vi "Part 2.vi"(11 "Input":string) -> (3 "Output":i64)   [LabVIEW 2021]
uses:
  3dc34be2-a6d3-4b17-bbb5-65f4369eede6.vi
  <userlib>/_OpenG.lib/string/string.llb/Convert EOLs (String)__ogtk.vi
panel:
  out "Array":bool[][](array[boolean])
  out "Grid":string[][](array[string])
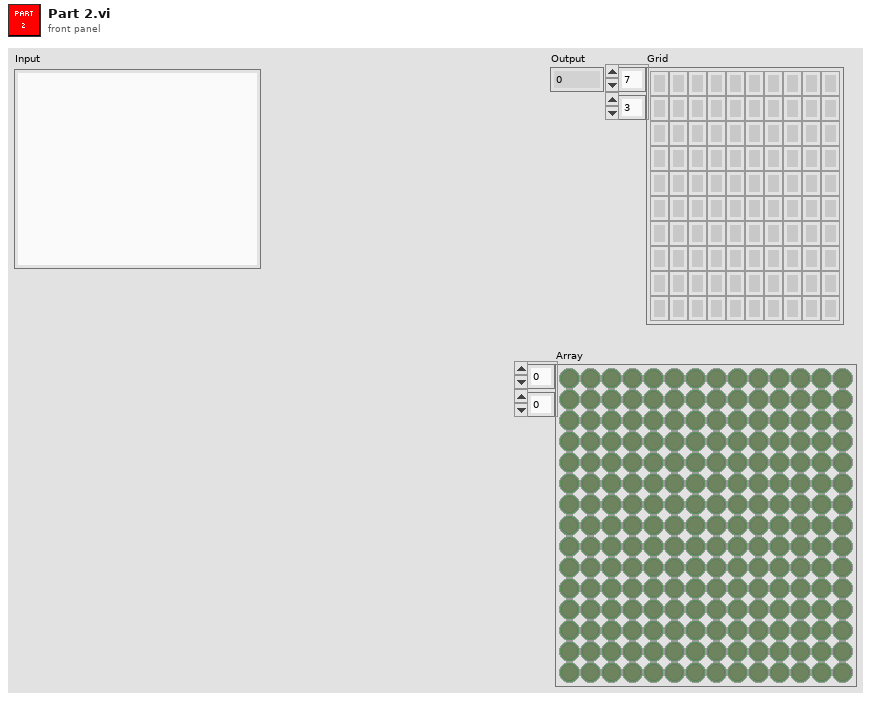
[diagram p1: front panel]
types:
  T1 = set{cluster{"row":i32, "col":i32, "dir":enum16{"right", "left", "up", "down"}}}
  T2 = cluster{"row":i32, "col":i32, "dir":enum16{"right", "left", "up", "down"}}[]
  T3 = cluster{"row":i32, "col":i32, "dir":enum16{"right", "left", "up", "down"}}
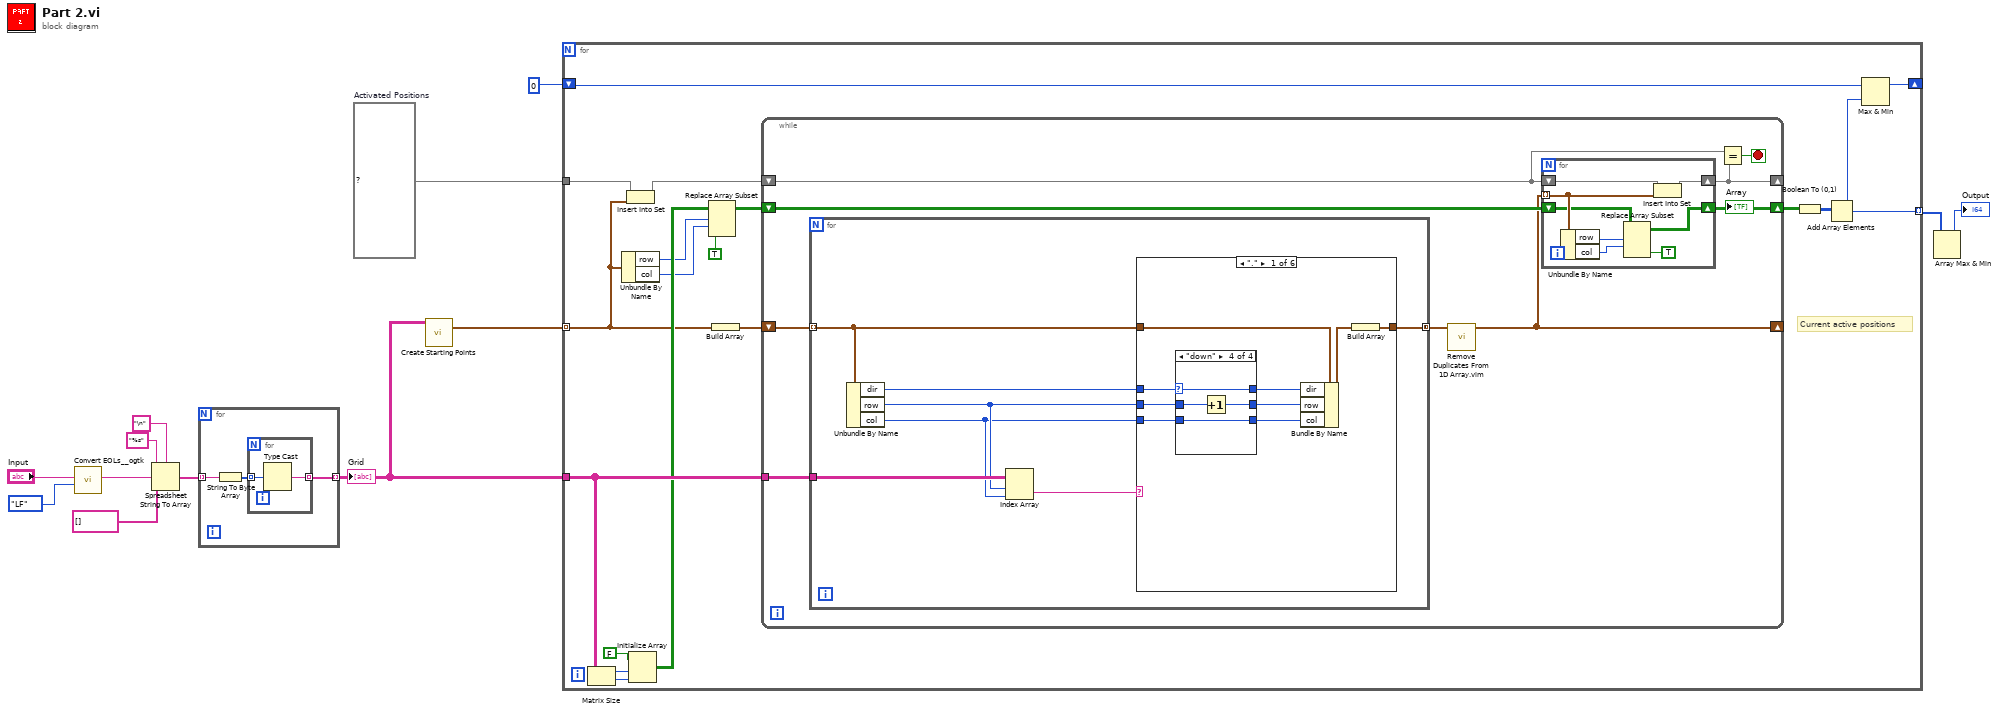
[diagram p0: block diagram]
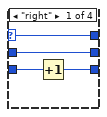
[diagram p2: hidden frame]
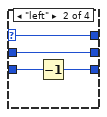
[diagram p3: hidden frame]
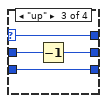
[diagram p4: hidden frame]
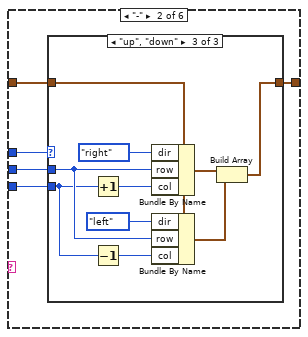
[diagram p5: hidden frame]
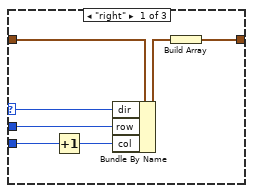
[diagram p6: hidden frame]
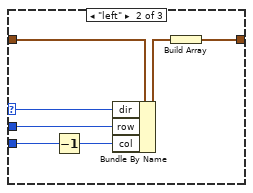
[diagram p7: hidden frame]
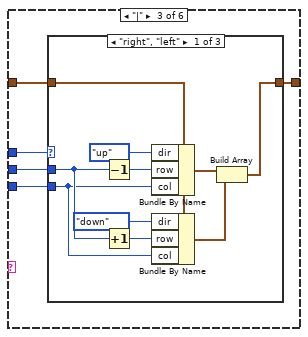
[diagram p8: hidden frame]
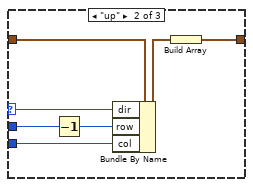
[diagram p9: hidden frame]
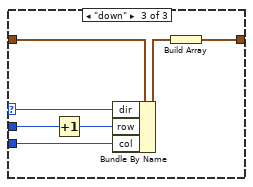
[diagram p10: hidden frame]
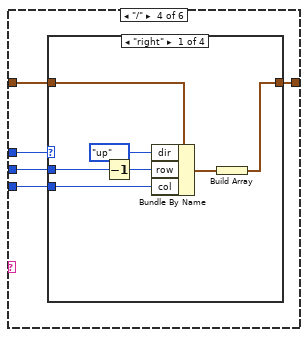
[diagram p11: hidden frame]
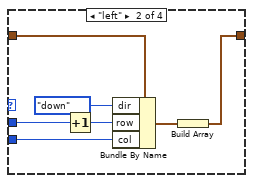
[diagram p12: hidden frame]
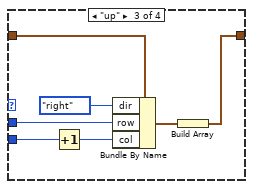
[diagram p13: hidden frame]
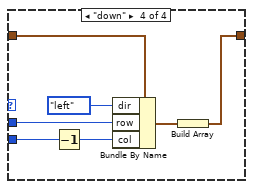
[diagram p14: hidden frame]
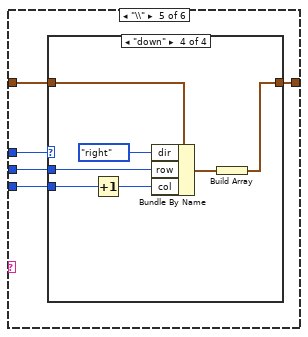
[diagram p15: hidden frame]
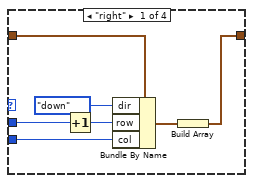
[diagram p16: hidden frame]
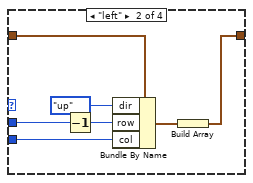
[diagram p17: hidden frame]
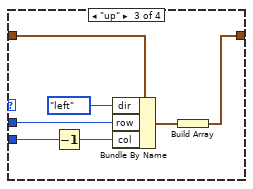
[diagram p18: hidden frame]
diagram:
  w6 = T1 {}  # Activated Positions
  n1 = call-poly <userlib>:"Convert EOLs__ogtk.vi"("Convert to:"=enum16{"CR", "LF", "CRLF"}."LF", "String in"="Input") -> ("String out"=w9:string)  [unwired: 9 in]
  n2 = Spreadsheet String To Array(delimiter (Tab)="\n", format string="%s", spreadsheet string=w9, array type (2D Dbl)=string[] []) -> (array=w7:string[])
  n3 = for {
    tunnel: w7 -> [w16] mode=indexing
    tunnel: [w14] -> w3 mode=indexing
    n4 = String To Byte Array(string=w16) -> (unsigned byte array=w15:u8[])
    n5 = for {
      tunnel: w15 -> [w18] mode=indexing
      tunnel: [w17] -> w14 mode=indexing
      n6 = Type Cast(x=w18) -> (*(type *) &x=w17:string)  [unwired: 1 in]
    }
  }
  "Grid" <- w3
  n7 = call "Create Starting Points.vi"("Grid"=w3) -> ("Starting Points"=w2:T2)  [unwired: 10 in]
  n8 = for {
    tunnel: w6 -> [w35]
    tunnel: w2 -> [w24] mode=indexing
    tunnel: w3 -> [w32]
    tunnel: [w19] -> w5 mode=indexing
    shift-right: [w21] -> _
    shift-left: 0 -> [w20]
    # "Current active positions"
    n9 = Matrix Size(0:w32) -> (1:w33:i32, 2:w31:i32)
    n10 = Unbundle By Name(w24) -> ("row"=w23:i32, "col"=w22:i32)
    n11 = Insert Into Set(10:w24, 11:w35) -> (3:w34:T1)  [unwired: 1 out]
    n12 = Initialize Array(FALSE, w33, w31) -> (w29:bool[][])
    n13 = Replace Array Subset(array=w29, new element=TRUE, index (row)=w23, index (col)=w22) -> (w28:bool[][])
    n14 = Build Array(w24) -> (w36:T2)
    n15 = while {
      shift-right: [w44] -> _
      shift-left: w34 -> [w43]
      shift-right: [w37] -> _
      shift-left: w36 -> [w42]
      tunnel: w32 -> [w40]
      shift-right: [w38] -> w26
      shift-left: w28 -> [w39]
      stop <- w45 stop-if-true
      n16 = for {
        tunnel: w42 -> [w49] mode=indexing
        tunnel: [w50] -> w41 mode=concatenating
        tunnel: w40 -> [w52]
        n17 = Unbundle By Name(w49) -> ("dir"=w48:enum16{"right", "left", "up", "down"}, "row"=w47:i32, "col"=w46:i32)
        n18 = Index Array(array=w52, index (row)=w47, index (col)=w46) -> (element=w51:string)
        n19 = case shown="\".\"" w51 {
          tunnel: w47 -> [w57 w80 w109 w138 w171 _]
          tunnel: w46 -> [w55 w79 w108 w137 w170 _]
          tunnel: w48 -> [w58 w81 w110 w139 w172 _]
          tunnel: w49 -> [w61 w82 w111 w140 w173 _]
          tunnel: [w60 w78 w107 w136 w169 _] -> w50
          frame "." {
            n20 = case shown="\"down\"" w58 {
              selector: w58 -> [w62 w66 w70 w74]
              tunnel: w57 -> [w65 w69 w72 w76]
              tunnel: w55 -> [w64 w68 w73 w77]
              tunnel: [w65 w69 w71 w75] -> w54
              tunnel: [w63 w67 w73 w77] -> w56
              tunnel: [w62 w66 w70 w74] -> w53
              frame "right" {
                n21 = Increment(x=w64) -> (x+1=w63:i32)
              }
              frame "left" {
                n22 = Decrement(x=w68) -> (x-1=w67:i32)
              }
              frame "up" {
                n23 = Decrement(x=w72) -> (x-1=w71:i32)
              }
              frame "down" {
                n24 = Increment(x=w76) -> (x+1=w75:i32)
              }
            }
            n25 = Bundle By Name(cluster=w61, "dir"=w53, "row"=w54, "col"=w56) -> (w59:T3)
            n26 = Build Array(w59) -> (w60:T2)
          }
          frame "-" {
            n27 = case shown="\"up\", \"down\"" w81 {
              selector: w81 -> [w88 w95 _]
              tunnel: w82 -> [w89 w96 w98]
              tunnel: w80 -> [w87 w94 w100]
              tunnel: w79 -> [w86 w93 w99]
              tunnel: [w84 w91 w106] -> w78
              frame "right" {
                n28 = Increment(x=w86) -> (x+1=w83:i32)
                n29 = Bundle By Name(cluster=w89, "dir"=w88, "row"=w87, "col"=w83) -> (w85:T3)
                n30 = Build Array(w85) -> (w84:T2)
              }
              frame "left" {
                n31 = Decrement(x=w93) -> (x-1=w90:i32)
                n32 = Bundle By Name(cluster=w96, "dir"=w95, "row"=w94, "col"=w90) -> (w92:T3)
                n33 = Build Array(w92) -> (w91:T2)
              }
              frame "up", "down" {
                n34 = Increment(x=w99) -> (x+1=w104:i32)
                n35 = Decrement(x=w99) -> (x-1=w103:i32)
                n36 = Bundle By Name(cluster=w98, "dir"=enum16{"right", "left", "up", "down"}."right", "row"=w100, "col"=w104) -> (w101:T3)
                n37 = Bundle By Name(cluster=w98, "dir"=enum16{"right", "left", "up", "down"}."left", "row"=w100, "col"=w103) -> (w97:T3)
                n38 = Build Array(w101, w97) -> (w106:T2)
              }
            }
          }
          frame "|" {
            n39 = case shown="\"right\", \"left\"" w110 {
              selector: w110 -> [_ w127 w134]
              tunnel: w111 -> [w115 w128 w135]
              tunnel: w109 -> [w117 w126 w133]
              tunnel: w108 -> [w116 w125 w132]
              tunnel: [w121 w123 w130] -> w107
              frame "right", "left" {
                n40 = Decrement(x=w117) -> (x-1=w113:i32)
                n41 = Increment(x=w117) -> (x+1=w112:i32)
                n42 = Bundle By Name(cluster=w115, "dir"=enum16{"right", "left", "up", "down"}."up", "row"=w113, "col"=w116) -> (w118:T3)
                n43 = Bundle By Name(cluster=w115, "dir"=enum16{"right", "left", "up", "down"}."down", "row"=w112, "col"=w116) -> (w114:T3)
                n44 = Build Array(w118, w114) -> (w121:T2)
              }
              frame "up" {
                n45 = Decrement(x=w126) -> (x-1=w122:i32)
                n46 = Bundle By Name(cluster=w128, "dir"=w127, "row"=w122, "col"=w125) -> (w124:T3)
                n47 = Build Array(w124) -> (w123:T2)
              }
              frame "down" {
                n48 = Increment(x=w133) -> (x+1=w129:i32)
                n49 = Bundle By Name(cluster=w135, "dir"=w134, "row"=w129, "col"=w132) -> (w131:T3)
                n50 = Build Array(w131) -> (w130:T2)
              }
            }
          }
          frame "/" {
            n51 = case shown="\"right\"" w139 {
              tunnel: w140 -> [w142 w149 w156 w163]
              tunnel: w138 -> [w144 w151 w158 w165]
              tunnel: w137 -> [w143 w150 w157 w164]
              tunnel: [w147 w154 w161 w168] -> w136
              frame "right" {
                n52 = Decrement(x=w144) -> (x-1=w141:i32)
                n53 = Bundle By Name(cluster=w142, "dir"=enum16{"right", "left", "up", "down"}."up", "row"=w141, "col"=w143) -> (w145:T3)
                n54 = Build Array(w145) -> (w147:T2)
              }
              frame "left" {
                n55 = Increment(x=w151) -> (x+1=w148:i32)
                n56 = Bundle By Name(cluster=w149, "dir"=enum16{"right", "left", "up", "down"}."down", "row"=w148, "col"=w150) -> (w152:T3)
                n57 = Build Array(w152) -> (w154:T2)
              }
              frame "up" {
                n58 = Increment(x=w157) -> (x+1=w155:i32)
                n59 = Bundle By Name(cluster=w156, "dir"=enum16{"right", "left", "up", "down"}."right", "row"=w158, "col"=w155) -> (w159:T3)
                n60 = Build Array(w159) -> (w161:T2)
              }
              frame "down" {
                n61 = Decrement(x=w164) -> (x-1=w162:i32)
                n62 = Bundle By Name(cluster=w163, "dir"=enum16{"right", "left", "up", "down"}."left", "row"=w165, "col"=w162) -> (w166:T3)
                n63 = Build Array(w166) -> (w168:T2)
              }
            }
          }
          frame "\\" {
            n64 = case shown="\"down\"" w172 {
              tunnel: w173 -> [w175 w182 w189 w196]
              tunnel: w171 -> [w177 w184 w191 w198]
              tunnel: w170 -> [w176 w183 w190 w197]
              tunnel: [w180 w187 w194 w201] -> w169
              frame "right" {
                n65 = Increment(x=w177) -> (x+1=w174:i32)
                n66 = Bundle By Name(cluster=w175, "dir"=enum16{"right", "left", "up", "down"}."down", "row"=w174, "col"=w176) -> (w178:T3)
                n67 = Build Array(w178) -> (w180:T2)
              }
              frame "left" {
                n68 = Decrement(x=w184) -> (x-1=w181:i32)
                n69 = Bundle By Name(cluster=w182, "dir"=enum16{"right", "left", "up", "down"}."up", "row"=w181, "col"=w183) -> (w185:T3)
                n70 = Build Array(w185) -> (w187:T2)
              }
              frame "up" {
                n71 = Decrement(x=w190) -> (x-1=w188:i32)
                n72 = Bundle By Name(cluster=w189, "dir"=enum16{"right", "left", "up", "down"}."left", "row"=w191, "col"=w188) -> (w192:T3)
                n73 = Build Array(w192) -> (w194:T2)
              }
              frame "down" {
                n74 = Increment(x=w197) -> (x+1=w195:i32)
                n75 = Bundle By Name(cluster=w196, "dir"=enum16{"right", "left", "up", "down"}."right", "row"=w198, "col"=w195) -> (w199:T3)
                n76 = Build Array(w199) -> (w201:T2)
              }
            }
          }
          frame "", Default {
          }
        }
      }
      n77 = call "Remove Duplicates From 1D Array.vim"("array"=w41) -> ("array with duplicates removed"=w37:T2)  [unwired: 10 in]
      n78 = for {
        shift-right: [w208] -> w44
        shift-left: w43 -> [w209]
        tunnel: w37 -> [w207] mode=indexing
        shift-right: [w203] -> w38
        shift-left: w39 -> [w205]
        n79 = Unbundle By Name(w207) -> ("row"=w206:i32, "col"=w204:i32)
        n80 = Replace Array Subset(array=w205, new element=TRUE, index (row)=w206, index (col)=w204) -> (w203:bool[][])
        n81 = Insert Into Set(10:w207, 11:w209) -> (3:w208:T1)  [unwired: 1 out]
      }
      "Array" <- w38
      n82 = Equal?(x=w43, y=w44) -> (x = y?=w45:bool)
    }
    n83 = Boolean To (0,1)(Boolean=w26) -> (0, 1=w25:i16[][])
    n84 = Add Array Elements(numeric array=w25) -> (sum=w19:i16)
    n85 = Max & Min(x=w20, y=w19) -> (max(x,y)=w21:i32)  [unwired: 1 out]
  }
  n86 = Array Max & Min(array=w5) -> (max value=→"Output":i16)  [unwired: 3 out]
